vi "VI Tester Project API Get Method Path.vi"(8 "error in (no error)":errorcluster, 11 "Project API Method":T1) -> (0 "error out":errorcluster, 2 "Path to VI Tester Project API Proxy VI":path)   [LabVIEW 2013]
uses:
  VI Tester Project API Method Selector - Enum.ctl
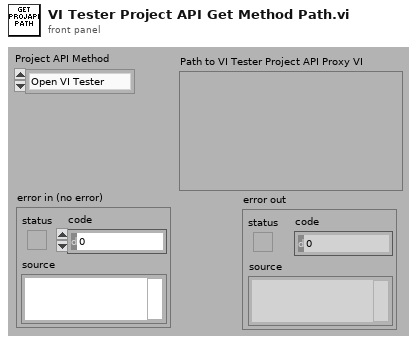
[diagram p1: front panel]
types:
  T1 = typedef "VI Tester Project API Method Selector - Enum.ctl" = enum16{"Open VI Tester", "Run All Tests", "Create New TestCase", "Create New TestSuite"}
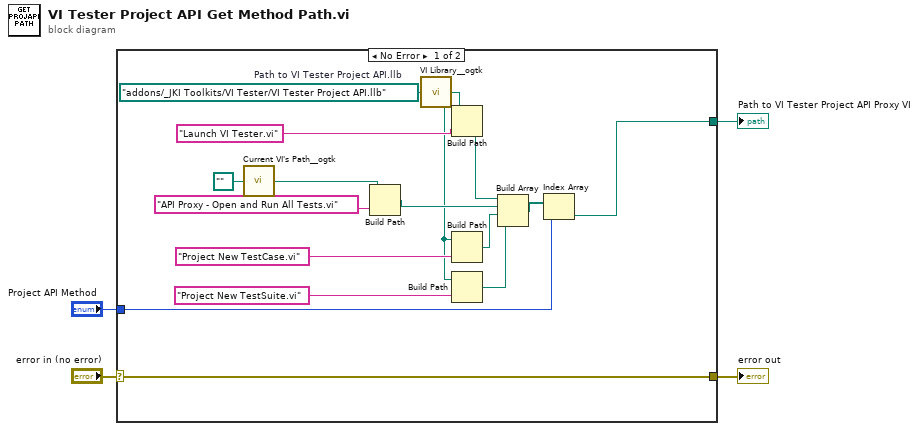
[diagram p0: block diagram]
diagram:
  n1 = case shown="No Error" "error in (no error)" {
    selector: "error in (no error)" -> [w18 w21]
    tunnel: "Project API Method" -> [w19 _]
    tunnel: [w16 _] -> w1
    tunnel: [w18 w21] -> w2
    frame No Error {
      w17 = path "addons/_JKI Toolkits/VI Tester/VI Tester Project API.llb"  # Path to VI Tester Project API.llb
      n2 = call <userlib>:"Current VI's Path__ogtk.vi"("Relative path (.)"=path "..") -> ("Current VI's Path (+ Relative)"=w11:path)
      n3 = Build Path(base path=w11, name or relative path="API Proxy - Open and Run All Tests.vi") -> (appended path=w9:path)
      n4 = call <userlib>:"VI Library__ogtk.vi"("Relative path (.)"=w17) -> ("VI Library (+ Relative)"=w6:path)
      n5 = Build Path(base path=w6, name or relative path="Launch VI Tester.vi") -> (appended path=w14:path)
      n6 = Build Path(base path=w6, name or relative path="Project New TestCase.vi") -> (appended path=w8:path)
      n7 = Build Path(base path=w6, name or relative path="Project New TestSuite.vi") -> (appended path=w7:path)
      n8 = Build Array(w14, w9, w8, w7) -> (w20:path[])
      n9 = Index Array(array=w20, index=w19) -> (element=w16:path)
    }
    frame Error {
    }
  }
  "Path to VI Tester Project API Proxy VI" <- w1
  "error out" <- w2
